vi "Read Datagram from Port.vi"(8 "error in (no error)":errorcluster, 9 "timeout ms (25000)":i32=25000 format="%d ms", 10 "max size (548)":i32, 11 "UDP Transceiver in":refnum<class "UDP Transceiver.lvclass">) -> (0 "error out":errorcluster, 1 "timed out?":bool, 2 "data":string, 3 "UDP Transceiver out":refnum<class "UDP Transceiver.lvclass">, 4 "source port":u16, 6 "source address":u32)   [LabVIEW 2017, in "UDP.lvlib" / "UDP Transceiver.lvclass"]
uses:
  UDP Transceiver.lvclass
  UDP Transceiver.lvclass/UDP Transceiver.ctl
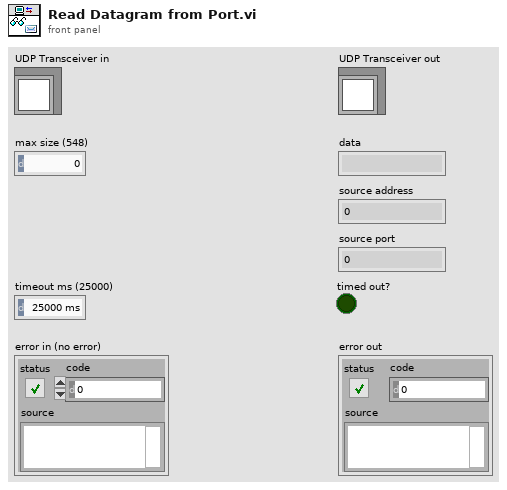
[diagram p1: front panel]
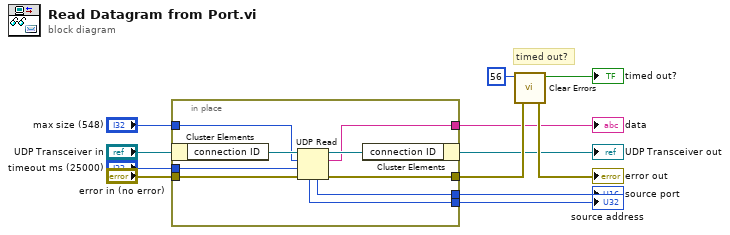
[diagram p0: block diagram]
diagram:
  # "timed out?"
  n1 = in-place {
    in-place-border: "error in (no error)" -> [w21]
    in-place-border: [w19] -> w11
    in-place-border: [w17] -> w8
    in-place-border: [w16] -> w7
    in-place-border: [w15] -> w9
    in-place-border: "max size (548)" -> [w14]
    in-place-border: "timeout ms (25000)" -> [w13]
    n2 = in-place-cluster #1("UDP Transceiver in") -> ("connection ID"=w18:refnum<k16>)
    n3 = UDP Read(connection ID=w18, max size (548)=w14, timeout ms (25000)=w13, 8:w21) -> (data out=w15:string, error out=w19:errorcluster, 3:w20:refnum<k16>, 4:w16:u16, 6:w17:u32)
    n4 = in-place-cluster #1("connection ID"=w20) -> (→"UDP Transceiver out":refnum<class "UDP Transceiver.lvclass">)
  }
  "data" <- w9
  "source address" <- w8
  "source port" <- w7
  n5 = call <vilib>:"Clear Errors.vi"("error in (no error)"=w11, "specific error code to clear (0: all)"=56) -> ("error out"=→"error out":errorcluster, "specific error cleared?"=→"timed out?":bool)  [unwired: 4 in]
